vi "Dependency to JSON.vi"(11 "Dependency":T1) -> (3 "Dependency JSON":string)   [LabVIEW 2020, in "neg-pkg.lvlib" / "Package.lvclass"]
uses:
  Package.lvclass
  Dependency.ctl
  Package ID.ctl
  Package Type.ctl
  neg_pkgs/negentropicdev/lv-json/JSON/JSON.lvlib
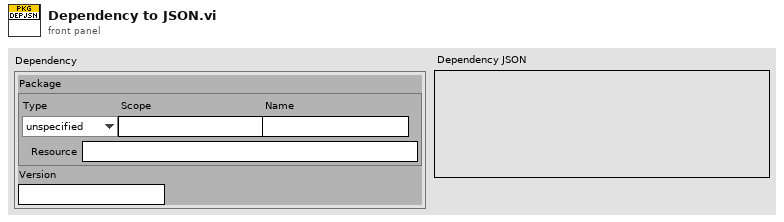
[diagram p1: front panel]
types:
  T1 = typedef "neg-pkg.lvlib/Package.lvclass/Dependency.ctl" = cluster{"Package":T2, "Version":string}
  T2 = typedef "neg-pkg.lvlib/Package.lvclass/Package ID.ctl" = cluster{"Type":T3, "Scope":string, "Name":string, "Resource":string}
  T3 = typedef "neg-pkg.lvlib/Package.lvclass/Package Type.ctl" = enum16{"unspecified", "git"}
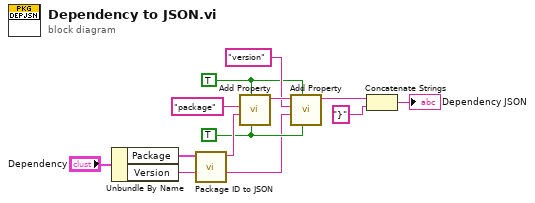
[diagram p0: block diagram]
diagram:
  w2 = TRUE
  w6 = TRUE
  n1 = Unbundle By Name("Dependency") -> ("Package"=w11:T2, "Version"=w1:string)
  n2 = call "Package ID to JSON.vi"("Package"=w11) -> ("Package JSON"=w10:string)  [unwired: 10 in]
  n3 = call "Add Property.vi"("String?"=w6, "Include Empty?"=w2, "Value"=w10, "Property Name"="package") -> ("String out"=w8:string)  [unwired: 7 in]
  n4 = call "Add Property.vi"("String?"=w6, "Include Empty?"=w2, "Value"=w1, "Property Name"="version", "String In"=w8) -> ("String out"=w5:string)  [unwired: 6 in]
  n5 = Concatenate Strings(w5, "}" ("string")) -> (→"Dependency JSON":string)
